vi "AxisFetchRegs.vi"(7 "read aditional data":bool, 8 "error in":errorcluster, 11 "Modbus master":refnum<class "Modbus Master.lvclass">) -> (0 "error out":errorcluster, 2 "JoyControl":T1 {"UnitsControl" items=["mm", "°"]}, 3 "AxisReadValues":T2)   [LabVIEW 2020, in "SMCD14_lib.lvlib"]
uses:
  SMCD14_lib.lvlib
  <vilib>/Modbus/master/Modbus Master.lvclass
  AxisReadValues_typedef.ctl
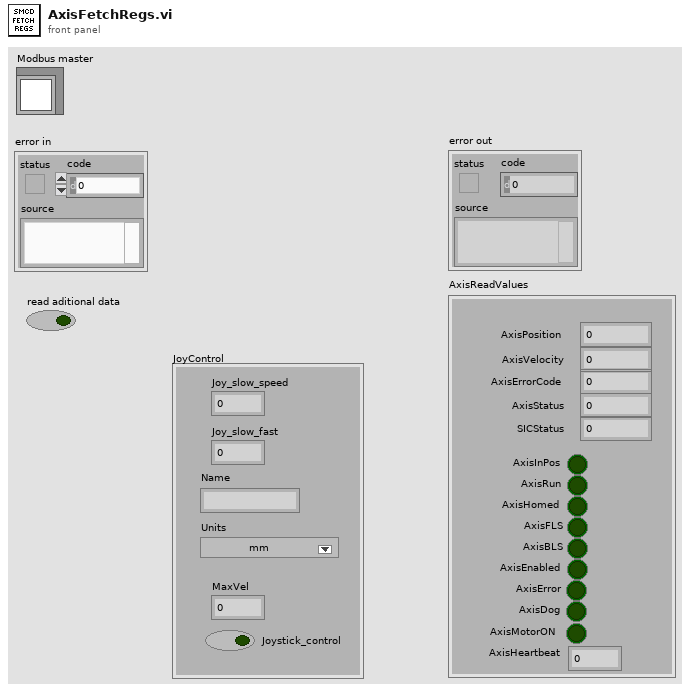
[diagram p1: front panel]
types:
  T1 = cluster{"Joy_slow_speed":sgl, "Joy_slow_fast":sgl, "Name":string, "UnitsControl":u16, "MaxVel":sgl, "Joystick_control":bool}
  T2 = typedef "SMCD14_lib.lvlib/AxisReadValues_typedef.ctl" = cluster{"AxisPosition":dbl, "AxisStatus":i16, "AxisErrorCode":i16, "AxisInPos":bool, "AxisRun":bool, "AxisHomed":bool, "AxisFLS":bool, "AxisBLS":bool, "AxisEnabled":bool, "AxisError":bool, "AxisDog":bool, "AxisVelocity":dbl, "AxisHeartbeat":i16, "SICStatus":i16, "AxisMotorON":bool}
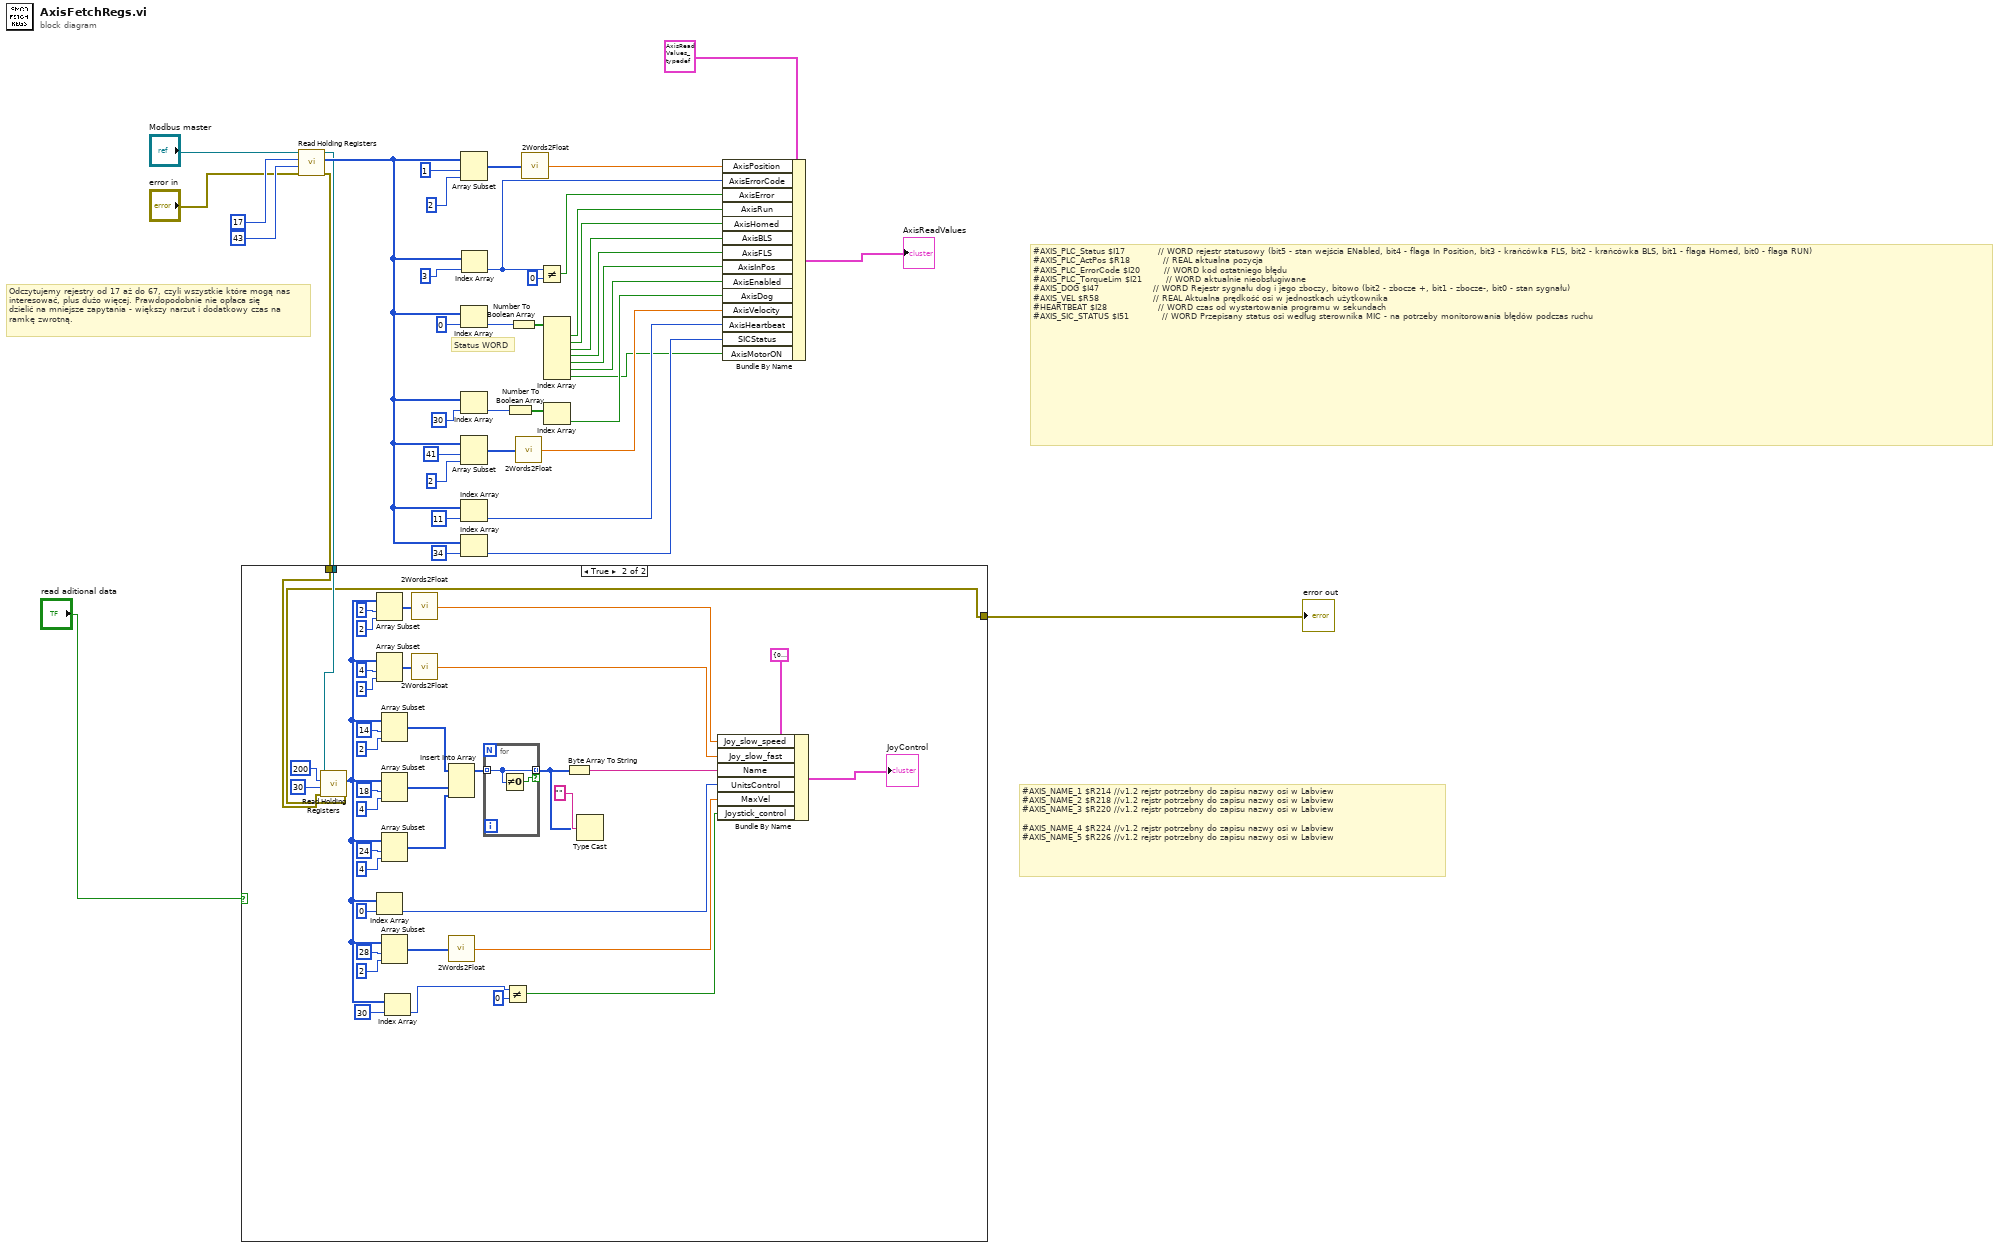
[diagram p0: block diagram]
diagram:
  # "#AXIS_NAME_1 $R214 //v1.2 rejstr potrzebny do zapisu nazwy osi w Labview\n#AXIS_NAME_2 $R218 //v1.2 rejstr potrzebny do zapisu nazwy osi w Labview\n#AXIS_NAME_3 $R220 //v1.2 rejstr potrzebny do zapisu nazwy osi w Labview\n\n#AXIS_NAME_4 $R224 //v1.2 rejstr potrzebny do zapisu nazwy osi w Labview\n#AXIS_NAME_5 $R226 //v1.2 rejstr potrzebny do zapisu nazwy osi w Labview"
  # "#AXIS_PLC_Status $I17           // WORD rejestr statusowy (bit5 - stan wejścia ENabled, bit4 - flaga In Position, bit3 - krańcówka FLS, bit2 - krańcówka BLS, bit1 - flaga Homed, bit0 - flaga RUN)\n#AXIS_PLC_ActPos $R18           // REAL aktualna pozycja\n#AXIS_PLC_ErrorCode $I20        // WORD kod ostatniego błędu\n#AXIS_PLC_TorqueLim $I21        // WORD aktualnie nieobsługiwane\n#AXIS_DOG $I47                  // WORD Rejestr sygnału dog i jego zboczy, bitowo (bit2 - zbocze +, bit1 - zbocze-, bit0 - stan sygnału) \n#AXIS_VEL $R58                  // REAL Aktualna prędkość osi w jednostkach użytkownika\n#HEARTBEAT $I28                 // WORD czas od wystartowania programu w sekundach\n#AXIS_SIC_STATUS $I51           // WORD Przepisany status osi według sterownika MIC - na potrzeby monitorowania błędów podczas ruchu"
  # "Status WORD"
  # "Odczytujemy rejestry od 17 aż do 67, czyli wszystkie które mogą nas\ninteresować, plus dużo więcej. Prawdopodobnie nie opłaca się\ndzielić na mniejsze zapytania - większy narzut i dodatkowy czas na\nramkę zwrotną."
  n1 = call-dynamic "Read Holding Registers.vi"("error in (no error)"="error in", "number of holding registers"=u16 43, "starting address"=u16 17, "Modbus master in"="Modbus master") -> ("error out"=w3:errorcluster, "register values"=w9:u16[], "Modbus master out"=w4:refnum<class "Modbus Master.lvclass">)  [unwired: 5 in]
  n2 = case shown="True" "read aditional data" {
    tunnel: w4 -> [_ w81]
    tunnel: w3 -> [w42 w80]
    tunnel: [w42 w79] -> w2
    frame False {
    }
    frame True {
      n3 = call-dynamic "Read Holding Registers.vi"("error in (no error)"=w80, "number of holding registers"=u16 30, "starting address"=u16 200, "Modbus master in"=w81) -> ("error out"=w79:errorcluster, "register values"=w47:u16[])  [unwired: 5 in, 1 out]
      n4 = Array Subset(array=w47, index=2, length=2) -> (w74:u16[])
      n5 = Array Subset(array=w47, index=4, length=2) -> (w70:u16[])
      n6 = Index Array(array=w47, index=0) -> (element=w66:u16)
      n7 = Array Subset(array=w47, index=14, length=2) -> (w55:u16[])
      n8 = Array Subset(array=w47, index=18, length=4) -> (w54:u16[])
      n9 = Array Subset(array=w47, index=24, length=4) -> (w53:u16[])
      n10 = Array Subset(array=w47, index=28, length=2) -> (w63:u16[])
      n11 = Index Array(array=w47, index=30) -> (element=w44:u16)
      n12 = call "2Words2Float.vi"("input"=w74) -> ("value"=w73:sgl)
      n13 = call "2Words2Float.vi"("input"=w70) -> ("value"=w69:sgl)
      n14 = Insert Into Array(array=w55, new element #1=w54, new element #2=w53) -> (w50:u16[])  [unwired: 1 in]
      n15 = call "2Words2Float.vi"("input"=w63) -> ("value"=w62:sgl)
      n16 = for {
        tunnel: w50 -> [w82] mode=indexing
        tunnel: [w82] -> w49 mode=indexing if=w83
        n17 = Not Equal To 0?(x=w82) -> (x != 0?=w83:bool)
      }
      n18 = Not Equal?(x=w44, y=u16 0) -> (x != y?=w43:bool)
      n19 = Byte Array To String(unsigned byte array=w49) -> (string=w51:string)
      n20 = Type Cast(type="", x=w49) -> ()  [unwired: 1 out]
      n21 = Bundle By Name(cluster=T1 {"Joy_slow_speed"=0.0, "Joy_slow_fast"=0.0, "Name"="", "UnitsControl"=0, "MaxVel"=0.0, "Joystick_control"=TRUE} ("Cluster"), "Joy_slow_speed"=w73, "Joy_slow_fast"=w69, "Name"=w51, "UnitsControl"=w66, "MaxVel"=w62, "Joystick_control"=w43) -> (→"JoyControl":T1)
    }
  }
  "error out" <- w2
  n22 = Array Subset(array=w9, index=1, length=2) -> (w36:u16[])
  n23 = Index Array(array=w9, index=0) -> (element=w33:u16)
  n24 = Index Array(array=w9, index=30) -> (element=w19:u16)
  n25 = Array Subset(array=w9, index=41, length=2) -> (w15:u16[])
  n26 = Index Array(array=w9, index=11) -> (element=w6:u16)
  n27 = Index Array(array=w9, index=34) -> (element=w7:u16)
  n28 = Index Array(array=w9, index=3 ("length")) -> (element=w30:u16)
  n29 = Number To Boolean Array(number=w19) -> (Boolean array=w20:bool[])
  n30 = Number To Boolean Array(number=w33) -> (Boolean array=w32:bool[])
  n31 = call "2Words2Float.vi"("input"=w15) -> ("value"=w14:sgl)
  n32 = call "2Words2Float.vi"("input"=w36) -> ("value"=w34:sgl)
  n33 = Not Equal?(x=w30, y=u16 0) -> (x != y?=w28:bool)
  n34 = Index Array(array=w32) -> (element #1=w27:bool, element #2=w26:bool, element #3=w25:bool, element #4=w24:bool, element #5=w23:bool, element #6=w22:bool, element #7=w5:bool)  [unwired: 7 in]
  n35 = Index Array(array=w20) -> (element=w18:bool)  [unwired: 1 in]
  n36 = Bundle By Name(cluster=T2 {"AxisPosition"=0.0, "AxisStatus"=0, "AxisErrorCode"=0, "AxisInPos"=FALSE, "AxisRun"=FALSE, "AxisHomed"=FALSE, "AxisFLS"=FALSE, "AxisBLS"=FALSE, "AxisEnabled"=FALSE, "AxisError"=FALSE, "AxisDog"=FALSE, "AxisVelocity"=0.0, "AxisHeartbeat"=0, "SICStatus"=0, "AxisMotorON"=FALSE} ("AxisReadValues"), "AxisPosition"=w34, "AxisErrorCode"=w30, "AxisError"=w28, "AxisRun"=w27, "AxisHomed"=w26, "AxisBLS"=w25, "AxisFLS"=w24, "AxisInPos"=w23, "AxisEnabled"=w22, "AxisDog"=w18, "AxisVelocity"=w14, "AxisHeartbeat"=w6, "SICStatus"=w7, "AxisMotorON"=w5) -> (→"AxisReadValues":T2)
